vi "ZeroMQ_WSTA.vi"() -> ()   [LabVIEW 2018]
uses:
  <vilib>/addons/zeromq/socket_type.ctl
  <vilib>/addons/zeromq/socket_options.ctl
  <vilib>/addons/zeromq/zeromq.lvlib
  <vilib>/addons/zeromq/zmq_socket.lvclass
  <vilib>/addons/zeromq/zmq_context.lvclass
panel:
  out "error out 4":errorcluster
  out "command":string
  in  "stop 3":bool
  out "error out 3":errorcluster
  out "error out 2":errorcluster
  out "message":string
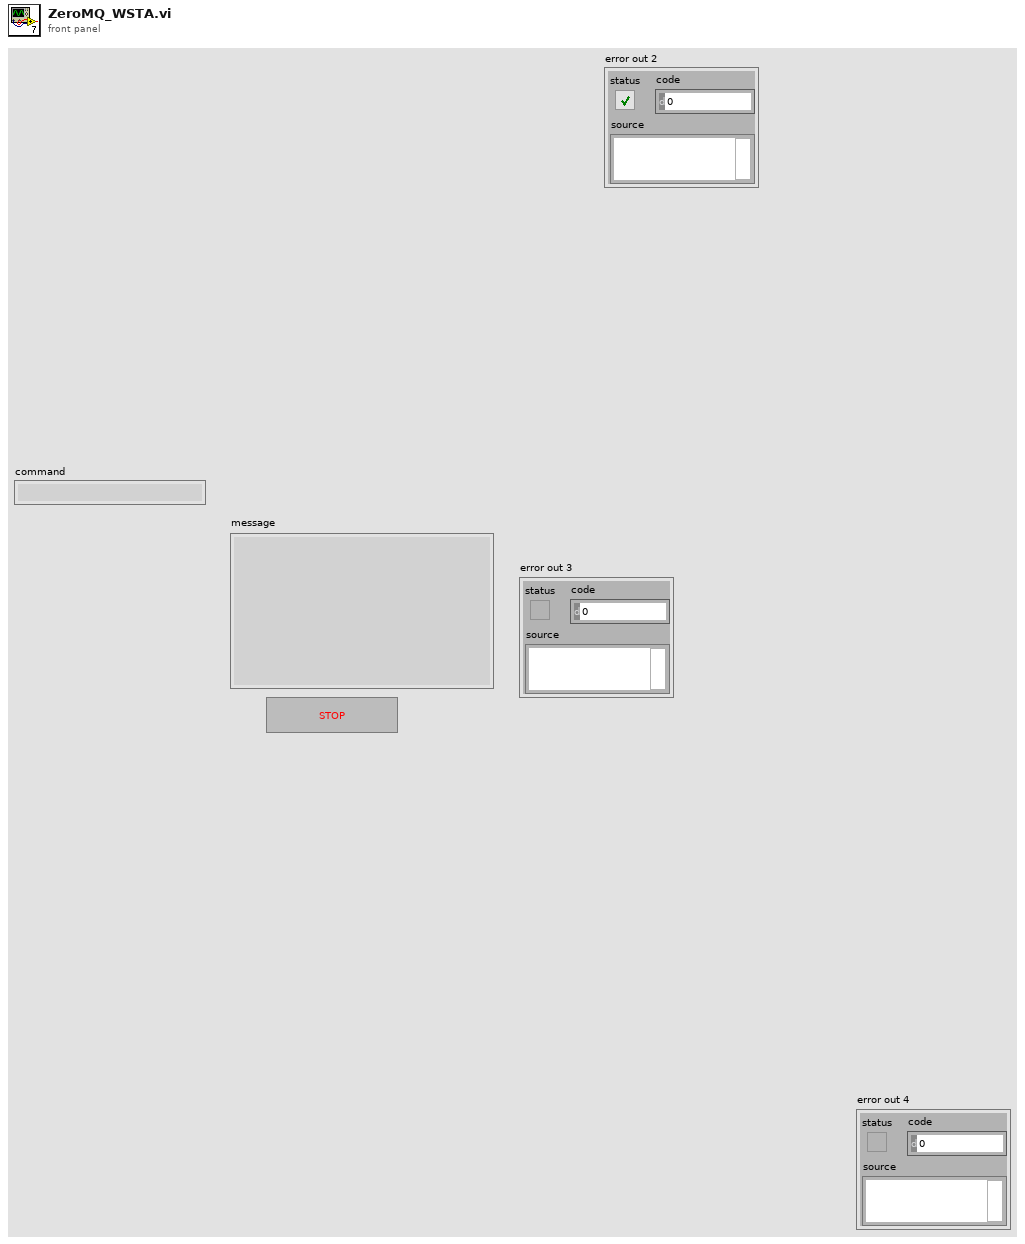
[diagram p1: front panel]
types:
  T1 = cluster{"ID":u32, "Address":string, "Service Name 1":string, "Service Name 2":string, "queue TX":refnum<queue>, "queue RX":refnum<queue>, "Port 1":u32, "Port 2":u32}
  T2 = typedef "zeromq.lvlib/socket_type.ctl" = enum8{"ZMQ_PAIR", "ZMQ_PUB", "ZMQ_SUB", "ZMQ_REQ", "ZMQ_REP", "ZMQ_DEALER", "ZMQ_ROUTER", "ZMQ_PULL", "ZMQ_PUSH", "ZMQ_XPUB", "ZMQ_XSUB", "ZMQ_STREAM", "ZMQ_SERVER", "ZMQ_CLIENT", "ZMQ_RADIO", "ZMQ_DISH", "ZMQ_GATHER", "ZMQ_SCATTER", "ZMQ_DGRAM"}
  T3 = typedef "zeromq.lvlib/socket_options.ctl" = enum8{"NONE", "ZMQ_HWM", "<2>", "ZMQ_SWAP", "ZMQ_AFFINITY", "ZMQ_ROUTING_ID", "ZMQ_SUBSCRIBE", "ZMQ_UNSUBSCRIBE", "ZMQ_RATE", "ZMQ_RECOVERY_IVL", "ZMQ_MCAST_LOOP", "ZMQ_SNDBUF", "ZMQ_RCVBUF", "ZMQ_RCVMORE", "ZMQ_FD", "ZMQ_EVENTS", "ZMQ_TYPE", "ZMQ_LINGER", "ZMQ_RECONNECT_IVL", "ZMQ_BACKLOG", "ZMQ_RECOVERY_IVL_MSEC", "ZMQ_RECONNECT_IVL_MAX", "ZMQ_MAXMSGSIZE", "ZMQ_SNDHWM", "ZMQ_RCVHWM", "ZMQ_MULTICAST_HOPS", "<26>", "ZMQ_RCVTIMEO", "ZMQ_SNDTIMEO", "<29>", "<30>", "ZMQ_IPV4ONLY", "ZMQ_LAST_ENDPOINT", "ZMQ_ROUTER_MANDATORY", "ZMQ_TCP_KEEPALIVE", "ZMQ_TCP_KEEPALIVE_CNT", "ZMQ_TCP_KEEPALIVE_IDLE", "ZMQ_TCP_KEEPALIVE_INTVL", "ZMQ_TCP_ACCEPT_FILTER", "ZMQ_IMMEDIATE", "ZMQ_XPUB_VERBOSE", "ZMQ_ROUTER_RAW", "ZMQ_IPV6", "ZMQ_MECHANISM", "ZMQ_PLAIN_SERVER", "ZMQ_PLAIN_USERNAME", "ZMQ_PLAIN_PASSWORD", "ZMQ_CURVE_SERVER", "ZMQ_CURVE_PUBLICKEY", "ZMQ_CURVE_SECRETKEY", "ZMQ_CURVE_SERVERKEY", "ZMQ_PROBE_ROUTER", "ZMQ_REQ_CORRELATE", "ZMQ_REQ_RELAXED", "ZMQ_CONFLATE", "ZMQ_ZAP_DOMAIN", "ZMQ_ROUTER_HANDOVER", "ZMQ_TOS", "ZMQ_IPC_FILTER_PID", "ZMQ_IPC_FILTER_UID", "ZMQ_IPC_FILTER_GID", "ZMQ_CONNECT_ROUTING_ID", "ZMQ_GSSAPI_SERVER", "ZMQ_GSSAPI_PRINCIPAL", "ZMQ_GSSAPI_SERVICE_PRINCIPAL", "ZMQ_GSSAPI_PLAINTEXT", "ZMQ_HANDSHAKE_IVL", "<67>", "ZMQ_SOCKS_PROXY", "ZMQ_XPUB_NODROP", "ZMQ_BLOCKY", "ZMQ_XPUB_MANUAL", "ZMQ_XPUB_WELCOME_MSG", "ZMQ_STREAM_NOTIFY", "ZMQ_INVERT_MATCHING", "ZMQ_HEARTBEAT_IVL", "ZMQ_HEARTBEAT_TTL", "ZMQ_HEARTBEAT_TIMEOUT", "ZMQ_XPUB_VERBOSER", "ZMQ_CONNECT_TIMEOUT", "ZMQ_TCP_MAXRT", "ZMQ_THREAD_SAFE", "<82>", "<83>", "ZMQ_MULTICAST_MAXTPDU", "ZMQ_VMCI_BUFFER_SIZE", "ZMQ_VMCI_BUFFER_MIN_SIZE", "ZMQ_VMCI_BUFFER_MAX_SIZE", "ZMQ_VMCI_CONNECT_TIMEOUT", "ZMQ_USE_FD", "ZMQ_GSSAPI_PRINCIPAL_NAMETYPE", "ZMQ_GSSAPI_SERVICE_PRINCIPAL_NAMETYPE", "ZMQ_BINDTODEVICE", "ZMQ_ZAP_ENFORCE_DOMAIN", "ZMQ_LOOPBACK_FASTPATH", "ZMQ_METADATA", "ZMQ_MULTICAST_LOOP", "ZMQ_ROUTER_NOTIFY"}
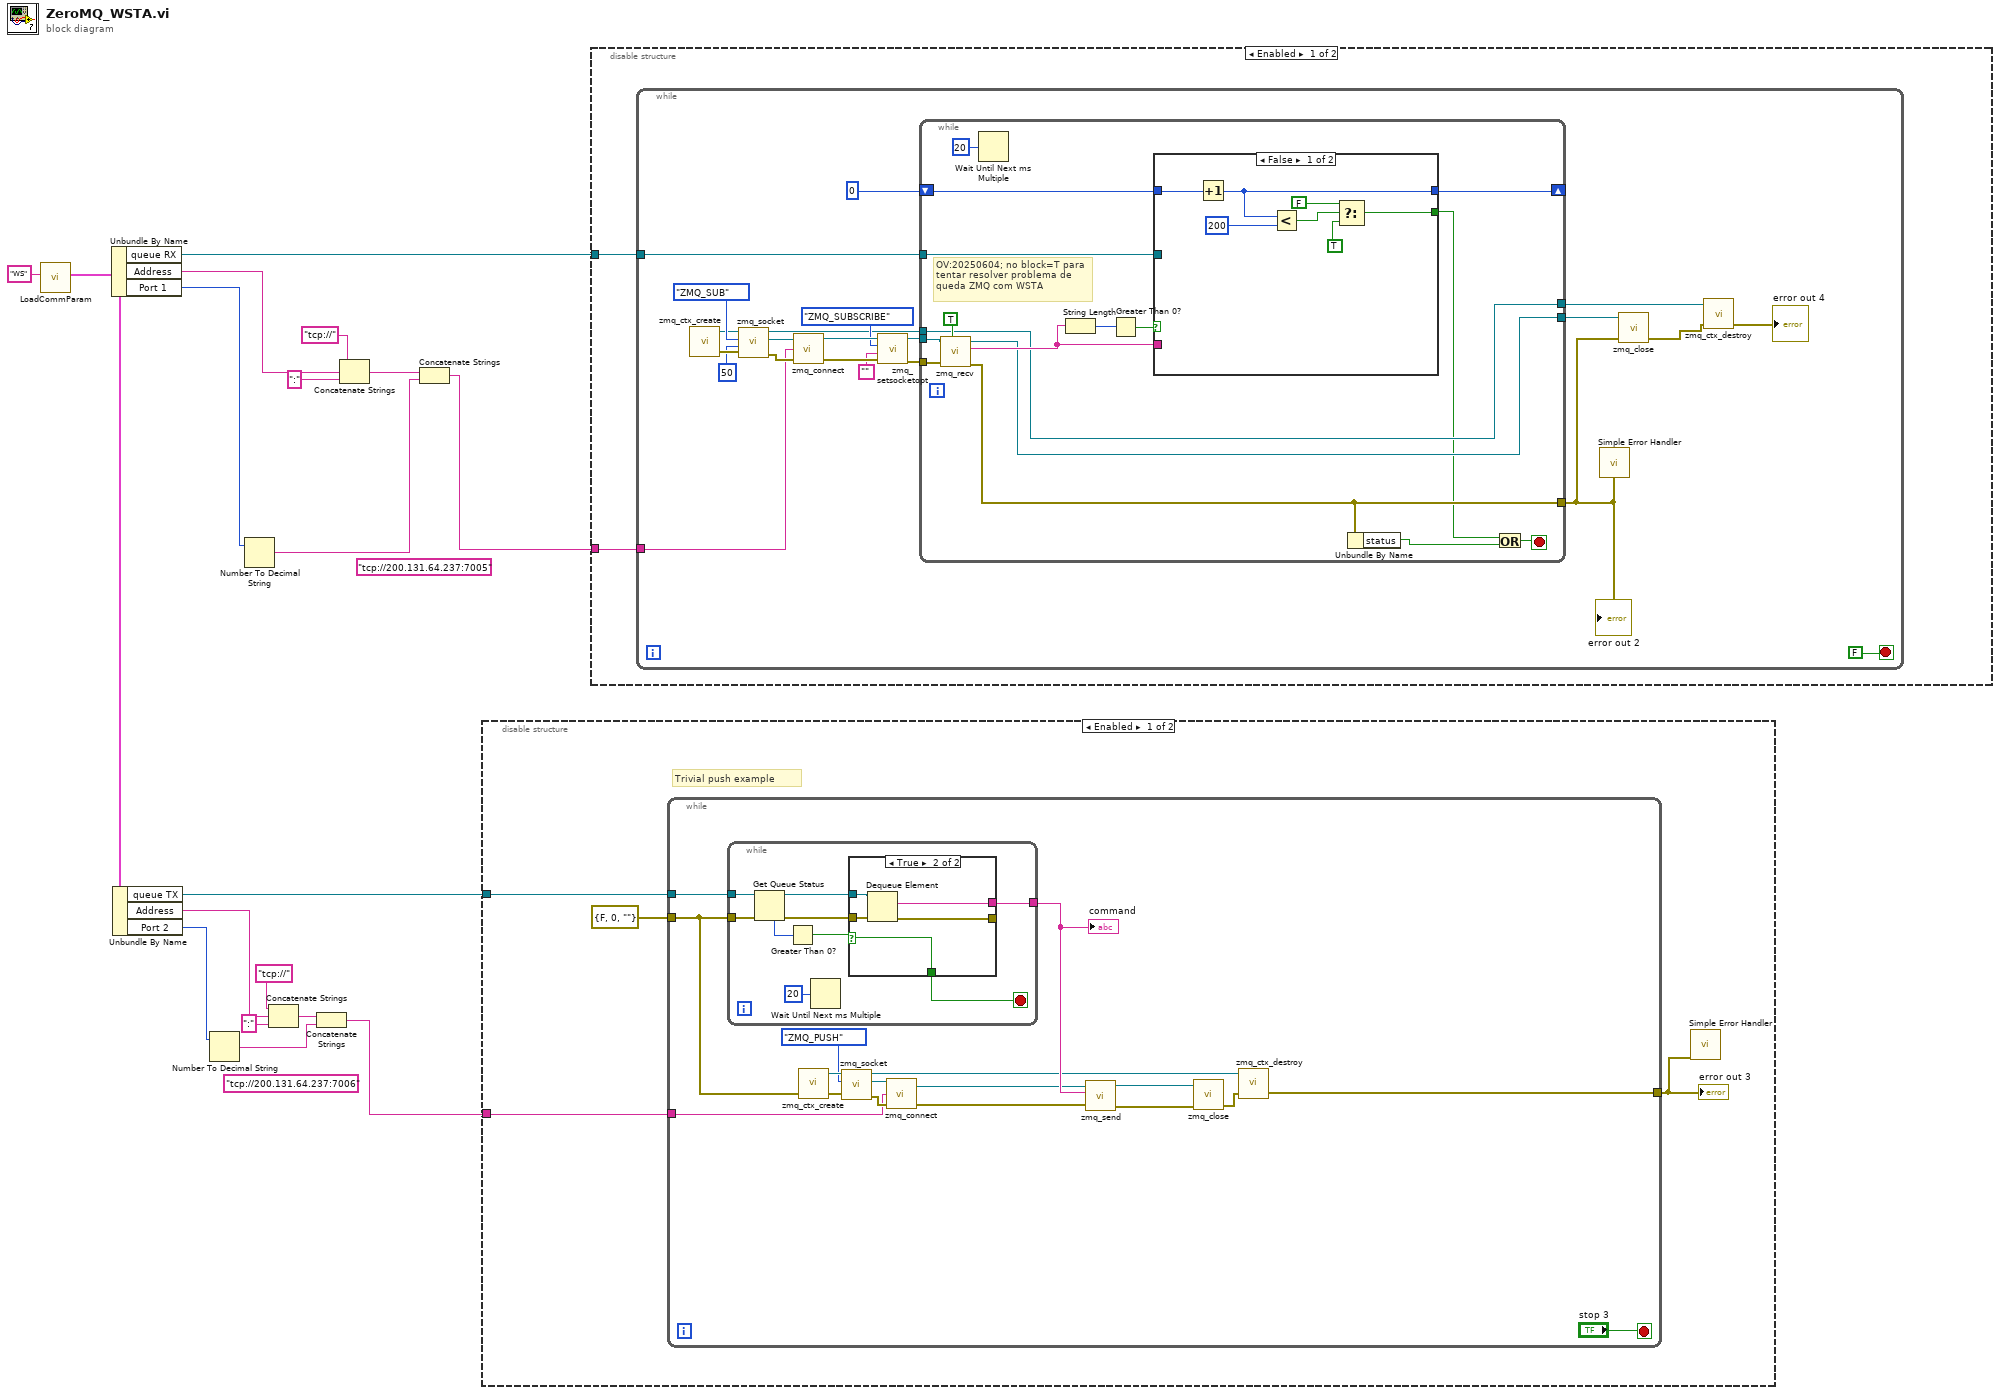
[diagram p0: block diagram]
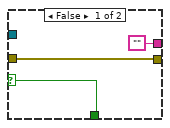
[diagram p2: hidden frame]
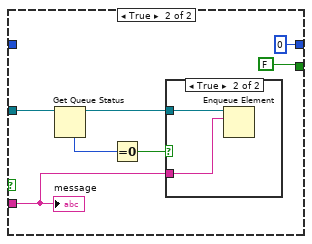
[diagram p4: hidden frame]
diagram:
  (unwired) "tcp://200.131.64.237:7006" ("endpoint")
  (unwired) "tcp://200.131.64.237:7005" ("endpoint")
  n1 = call "LoadCommParam.vi"("section name"="WS") -> ("output cluster"=w1:T1)  [unwired: 10 in]
  n2 = Unbundle By Name(w1) -> ("queue RX"=w5:refnum<queue>, "Address"=w17:string, "Port 1"=w16:u32)
  n3 = Unbundle By Name(w1) -> ("queue TX"=w3:refnum<queue>, "Address"=w7:string, "Port 2"=w6:u32)
  n4 = Number To Decimal String(number=w6) -> (decimal integer string=w11:string)  [unwired: 1 in]
  n5 = Number To Decimal String(number=w16) -> (decimal integer string=w15:string)  [unwired: 1 in]
  n6 = Concatenate Strings("tcp://" ("string"), w7, ":" ("string")) -> (w10:string)
  n7 = Concatenate Strings(w10, w11) -> (w2:string)
  n8 = Concatenate Strings("tcp://" ("string"), w17, ":" ("string")) -> (w14:string)
  n9 = Concatenate Strings(w14, w15) -> (w4:string)
  n10 = disable-structure shown="Enabled" {
    disable-tunnel: w3 -> [w21 _]
    disable-tunnel: w2 -> [w19 _]
    frame Enabled {
      # "Trivial push example"
      n11 = while {
        tunnel: w21 -> [w39]
        tunnel: errorcluster {"status"=FALSE, "code"=0, "source"=""} ("error out") -> [w24]
        tunnel: [w28] -> w22
        tunnel: w19 -> [w23]
        stop <- "stop 3" stop-if-true
        n12 = while {
          tunnel: w39 -> [w47]
          tunnel: w24 -> [w46]
          tunnel: [w42] -> w38
          stop <- w41 stop-if-true
          n13 = Get Queue Status(queue=w47, error in (no error)=w46) -> (queue out=w43:refnum<queue>, error out=w44:errorcluster, # elements in queue=w48:i32)  [unwired: 1 in, 5 out]
          n14 = Greater Than 0?(x=w48) -> (x > 0?=w45:bool)
          n15 = Wait Until Next ms Multiple(millisecond multiple=u32 20) -> ()  [unwired: 1 out]
          n16 = case shown="True" w45 {
            selector: w45 -> [w49 w52]
            tunnel: w44 -> [w51 w56]
            tunnel: w43 -> [_ w55]
            tunnel: [w51 w54] -> _
            tunnel: ["" w53] -> w42
            tunnel: [w49 w52] -> w41
            frame False {
            }
            frame True {
              n17 = Dequeue Element(queue=w55, error in (no error)=w56) -> (element=w53:string, error out=w54:errorcluster)  [unwired: 1 in, 2 out]
            }
          }
        }
        "command" <- w38
        n18 = call <vilib>:"zmq_ctx_create.vi"("error in"=w24) -> ("error out"=w33:errorcluster, "context out"=w36:refnum<class "zmq_context.lvclass">)  [unwired: 3 in]
        n19 = call <vilib>:"zmq_socket.vi"("error in"=w33, "socket type"=socket_type."ZMQ_PUSH", "context in"=w36) -> ("error out"=w35:errorcluster, "socket out"=w34:refnum<class "zmq_socket.lvclass">, "context out"=w27:refnum<class "zmq_context.lvclass">)  [unwired: 2 in]
        n20 = call <vilib>:"zmq_connect.vi"("error in"=w35, "endpoint"=w23, "socket in"=w34) -> ("error out"=w30:errorcluster, "socket out"=w31:refnum<class "zmq_socket.lvclass">)  [unwired: 1 in]
        n21 = call <vilib>:"zmq_send.vi"("error in"=w30, "data"=w38, "socket in"=w31) -> ("error out"=w25:errorcluster, "socket out"=w26:refnum<class "zmq_socket.lvclass">)  [unwired: 4 in]
        n22 = call <vilib>:"zmq_close.vi"("error in"=w25, "socket"=w26) -> ("error out"=w29:errorcluster)  [unwired: 3 in]
        n23 = call <vilib>:"zmq_ctx_destroy.vi"("error in"=w29, "context in"=w27) -> ("error out"=w28:errorcluster)  [unwired: 3 in]
      }
      "error out 3" <- w22
      n24 = call <vilib>:"Simple Error Handler.vi"("error in (no error)"=w22) -> ()  [unwired: 4 in, 5 out]
    }
    frame Disabled {
    }
  }
  n25 = disable-structure shown="Enabled" {
    disable-tunnel: w5 -> [w58 _]
    disable-tunnel: w4 -> [w57 _]
    frame Enabled {
      n26 = while {
        tunnel: w58 -> [w68]
        tunnel: w57 -> [w67]
        stop <- FALSE stop-if-true
        n27 = call <vilib>:"zmq_ctx_create.vi"() -> ("error out"=w79:errorcluster, "context out"=w70:refnum<class "zmq_context.lvclass">)  [unwired: 4 in]
        n28 = call <vilib>:"zmq_socket.vi"("error in"=w79, "linger (ms)"=50, "socket type"=socket_type."ZMQ_SUB", "context in"=w70) -> ("error out"=w78:errorcluster, "socket out"=w71:refnum<class "zmq_socket.lvclass">, "context out"=w62:refnum<class "zmq_context.lvclass">)  [unwired: 1 in]
        n29 = call <vilib>:"zmq_connect.vi"("error in"=w78, "endpoint"=w67, "socket in"=w71) -> ("error out"=w76:errorcluster, "socket out"=w77:refnum<class "zmq_socket.lvclass">)  [unwired: 1 in]
        n30 = call <vilib>:"zmq_setsocketopt.vi"("error in"=w76, "value"="", "option"=socket_options."ZMQ_SUBSCRIBE", "socket in"=w77) -> ("error out"=w75:errorcluster, "socket out"=w74:refnum<class "zmq_socket.lvclass">)  [unwired: 2 in]
        n31 = while {
          tunnel: w74 -> [w95]
          tunnel: w75 -> [w96]
          tunnel: [w88] -> w64
          tunnel: w68 -> [w92]
          tunnel: [w85] -> w63
          tunnel: w62 -> [w84]
          tunnel: [w84] -> w61
          shift-right: [w82] -> _
          shift-left: 0 ("linger (ms)") -> [w83]
          stop <- w86 stop-if-true
          # "OV:20250604; no block=T para\ntentar resolver problema de\nqueda ZMQ com WSTA"
          n32 = call <vilib>:"zmq_recv.vi"("no block? (F)"=TRUE, "error in"=w96, "socket in"=w95) -> ("error out"=w88:errorcluster, "data"=w91:string, "socket out"=w85:refnum<class "zmq_socket.lvclass">)  [unwired: 2 in, 2 out]
          n33 = Wait Until Next ms Multiple(millisecond multiple=u32 20) -> ()  [unwired: 1 out]
          n34 = String Length(string=w91) -> (length=w94:i32)
          n35 = Greater Than 0?(x=w94) -> (x > 0?=w93:bool)
          n36 = case shown="False" w93 {
            tunnel: w92 -> [_ w109]
            tunnel: w91 -> [_ w106]
            tunnel: w83 -> [w103 _]
            tunnel: [w102 0 ("linger (ms)")] -> w82
            tunnel: [w97 FALSE ("no block? (F)")] -> w81
            frame False {
              n37 = Increment(x=w103) -> (x+1=w102:i32)
              n38 = Less?(x=w102, y=200) -> (x < y?=w100:bool)
              n39 = Select(t=FALSE ("no block? (F)"), s=w100, f=TRUE ("no block? (F)")) -> (s? t:f=w97:bool)
            }
            frame True {
              n40 = Get Queue Status(queue=w109) -> (queue out=w107:refnum<queue>, # elements in queue=w110:i32)  [unwired: 2 in, 6 out]
              n41 = Equal To 0?(x=w110) -> (x = 0?=w108:bool)
              n42 = case shown="True" w108 {
                tunnel: w107 -> [_ w112]
                tunnel: w106 -> [_ w111]
                frame False {
                }
                frame True {
                  n43 = Enqueue Element(queue=w112, element=w111) -> ()  [unwired: 2 in, 3 out]
                }
              }
              "message" <- w106
            }
          }
          n44 = Unbundle By Name(w88) -> ("status"=w87:bool)
          n45 = Or(x=w81, y=w87) -> (x .or. y?=w86:bool)
        }
        "error out 2" <- w64
        n46 = call <vilib>:"Simple Error Handler.vi"("error in (no error)"=w64) -> ()  [unwired: 4 in, 5 out]
        n47 = call <vilib>:"zmq_close.vi"("error in"=w64, "socket"=w63) -> ("error out"=w66:errorcluster)  [unwired: 3 in]
        n48 = call <vilib>:"zmq_ctx_destroy.vi"("error in"=w66, "context in"=w61) -> ("error out"=→"error out 4":errorcluster)  [unwired: 3 in]
      }
    }
    frame Disabled {
    }
  }
